vi "errorHandlingDetails.vi"() -> ()   [LabVIEW 2014]
uses:
  <vilib>/Utility/error.llb/DialogType.ctl
panel:
  in  "Type of Error Dialog":T1=1 items=["no dialog", "OK message", "continue or stop message", "OK message + warnings", "continue/stop + warnings"]
  in  "Iteration to Issue Error":i32(knob) scale=0.0..5.0
  out "Combined Errors":errorcluster
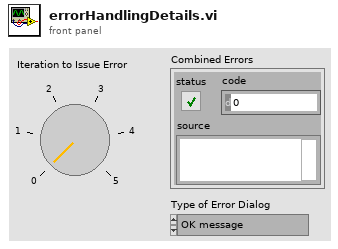
[diagram p1: front panel]
types:
  T1 = typedef "DialogType.ctl" = u16
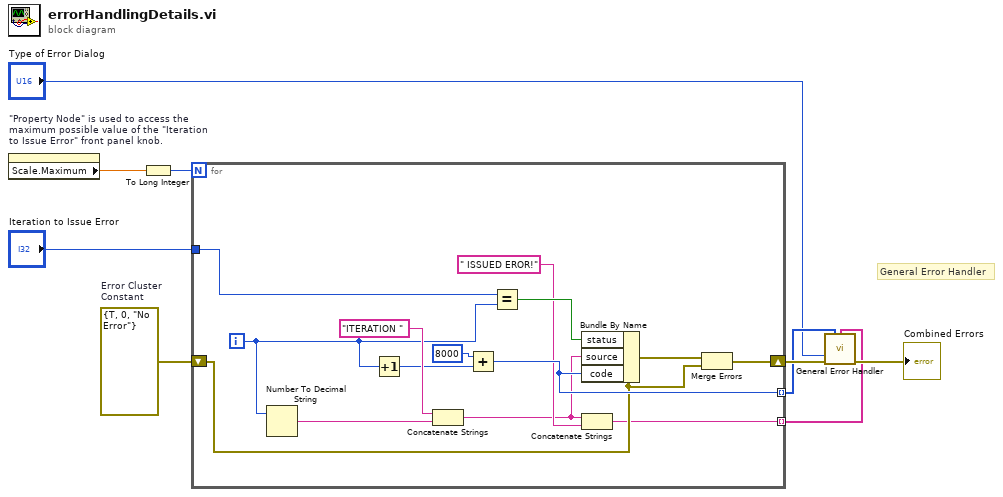
[diagram p0: block diagram]
diagram:
  w7 = errorcluster {"status"=TRUE, "code"=0, "source"="No Error"}  # Error Cluster  Constant
  # "General Error Handler"
  n1 = property on="\"Property Node\" is used to access the \nmaximum possible value of the \"Iteration \nto Issue Error\" front panel knob." class="Knob (strict)"() -> ("Scale.Maximum"=w6:dbl)  [unwired: 2 in, 2 out]
  n2 = To Long Integer(number=w6) -> (32bit integer=w2:i32)
  n3 = for {
    N: w2 -> [_]
    shift-right: [w21] -> w9
    shift-left: w7 -> [w13]
    tunnel: "Iteration to Issue Error" -> [w18]
    tunnel: [w16] -> w4 mode=indexing
    tunnel: [w10] -> w3 mode=indexing
    i -> [w15]
    n4 = Number To Decimal String(number=w15) -> (decimal integer string=w22:string)  [unwired: 1 in]
    n5 = Increment(x=w15) -> (x+1=w19:i32)
    n6 = Concatenate Strings "Concatenate Strings"("ITERATION ", w22) -> (w11:string)
    n7 = Add(x=8000, y=w19) -> (x+y=w16:i32)
    n8 = Equal?(x=w18, y=w15) -> (x = y?=w17:bool)
    n9 = Bundle By Name "Bundle By Name"(cluster=w13, "status"=w17, "source"=w11, "code"=w16) -> (w14:errorcluster)
    n10 = Concatenate Strings(w11, " ISSUED EROR!" ("string")) -> (w10:string)
    n11 = Merge Errors(w14, w13) -> (w21:errorcluster)
  }
  n12 = call <vilib>:"General Error Handler.vi"("[user-defined codes]"=w4, "[user-defined descriptions]"=w3, "type of dialog (OK msg:1)"="Type of Error Dialog", "error in (no error)"=w9) -> ("error out"=→"Combined Errors":errorcluster)  [unwired: 7 in, 4 out]
